vi "Device Write.vi"(4 "error in (no error)":errorcluster, 5 "Value":refnum<class "TTLControlledDevice.lvclass">, 6 "Container State":T3, 7 "Display State In":T1) -> (0 "error out":errorcluster, 3 "Display State Out":T1)   [LabVIEW 2015, in "TTLController.xctl"]
uses:
  TTLController.xctl
  <vilib>/_xctls/Container State.ctl
  Device Classes/Base Class/TTLControlledDevice.lvclass
  State.ctl
  Events.ctl
  Event Type.ctl
  Height Change.vi
  <vilib>/_xctls/XControlSupport.lvlib
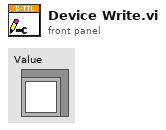
[diagram p1: front panel]
types:
  T1 = typedef "TTLController.xctl/State.ctl" = cluster{"Active":bool, "Device":refnum<class "TTLControlledDevice.lvclass">, "Events":T2, "Height":i32}
  T2 = typedef "TTLController.xctl/Events.ctl" = cluster{"Generic":refnum<user-event>, "Height":refnum<user-event>}
  T3 = typedef "XControlSupport.lvlib/Container State.ctl" = cluster{"Indicator?":bool, "Run Mode?":bool, " Refnum":refnum<vi>}
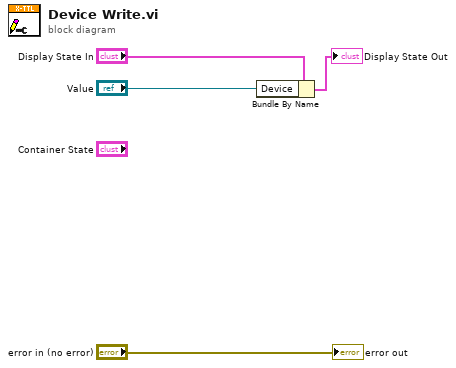
[diagram p0: block diagram]
diagram:
  n1 = Bundle By Name(cluster="Display State In", "Device"="Value") -> (→"Display State Out":T1)
  "error out" <- "error in (no error)"
